vi "dfd_FXP Interpolation Simu.vi"(0 "signal in":i64[](array[numeric]), 2 "PROD2SUM":i16, 3 "init?":bool, 5 "interpolation factor":i32, 9 "coef":i64[](array[numeric]), 11 "FXPMRateSimState in":T1, 12 "#taps per phase":i32) -> (4 "signal out":i64[](array[numeric]), 15 "FXPMRateSimState out":T1)   [LabVIEW 2017, in "NI_DigFilter_FXP.lvlib"]
uses:
  <vilib>/addons/Digital Filter Design/NI_DigFilter_FXP.lvlib
  <vilib>/addons/Digital Filter Design/_Objects.llb/dfd_FXP MRate Simu State.ctl
  <vilib>/addons/Digital Filter Design/_Objects.llb/dfd_Integer I160.ctl
  <vilib>/addons/Digital Filter Design/_Objects.llb/dfd_Index Config.ctl
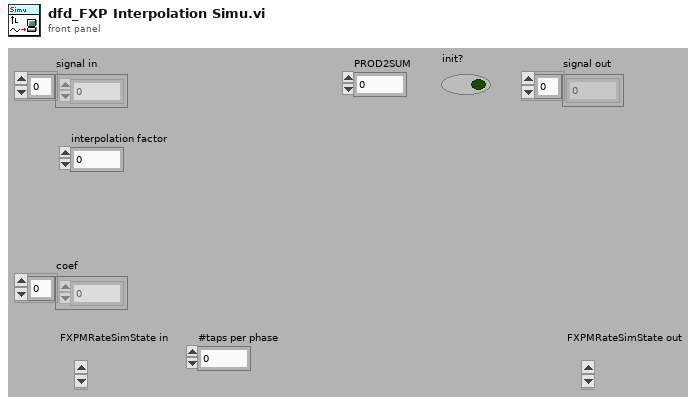
[diagram p1: front panel]
types:
  T1 = typedef "dfd_FXP MRate Simu State.ctl" = cluster{"acc1":T2[], "acc2":T2[], "FIR state":i64[], "next phase":i32}
  T2 = typedef "dfd_Integer I160.ctl" = cluster{"Hi [I32]":i32, "Lo3 [U32]":u32, "Lo2 [U32]":u32, "Lo1 [U32]":u32, "Lo0 [U32]":u32}
  T3 = typedef "dfd_Index Config.ctl" = cluster{"start":i32, "stepsize":i32}
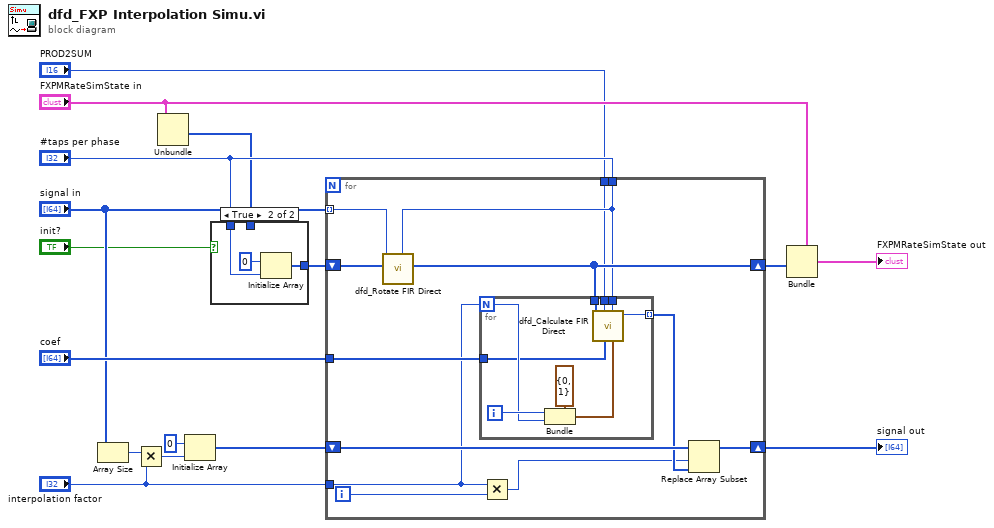
[diagram p0: block diagram]
diagram:
  n1 = Array Size(array="signal in") -> (size(s)=w11:i32)
  n2 = Multiply(x=w11, y="interpolation factor") -> (x*y=w14:i32)
  n3 = Unbundle("FXPMRateSimState in") -> ("FIR state"=w7:i64[])  [unwired: 3 out]
  n4 = Initialize Array(i64 0 ("element"), w14) -> (w12:i64[])
  n5 = case shown="True" "init?" {
    tunnel: [w17 w19] -> w8
    tunnel: "#taps per phase" -> [_ w18]
    tunnel: w7 -> [w17 _]
    frame False {
    }
    frame True {
      n6 = Initialize Array(i64 0 ("element"), w18) -> (w19:i64[])
    }
  }
  n7 = for {
    tunnel: "signal in" -> [w27] mode=indexing
    tunnel: "interpolation factor" -> [w23]
    tunnel: "#taps per phase" -> [w22]
    shift-right: [w24] -> w5
    shift-left: w8 -> [w26]
    tunnel: "coef" -> [w32]
    shift-right: [w28] -> w1
    shift-left: w12 -> [w30]
    tunnel: "PROD2SUM" -> [w21]
    i -> [w31]
    n8 = call <vilib>:"dfd_Rotate FIR Direct.vi"("#taps per phase"=w22, "state in"=w26, "x"=w27) -> ("state out"=w24:i64[])  [unwired: 1 in, 7 out]
    n9 = for {
      N: w23 -> [w35]
      tunnel: w22 -> [w38]
      tunnel: w24 -> [w36]
      tunnel: [w41] -> w29 mode=indexing
      tunnel: w32 -> [w34]
      tunnel: w21 -> [w33]
      i -> [w39]
      n10 = Bundle(cluster=T3 {"start"=0, "stepsize"=1} ("state idx"), "start"=w39, "stepsize"=w35) -> (w37:T3)
      n11 = call <vilib>:"dfd_Calculate FIR Direct.vi"("coef idx"=w37, "#taps per phase"=w38, "coef"=w34, "fwl_diff"=w33, "state in"=w36) -> ("y"=w41:i64)  [unwired: 3 in, 3 out]
    }
    n12 = Multiply(x=w23, y=w31) -> (x*y=w25:i32)
    n13 = Replace Array Subset(array=w30, new element=w29, index=w25) -> (w28:i64[])
  }
  "signal out" <- w1
  n14 = Bundle(cluster="FXPMRateSimState in", "FIR state"=w5) -> (→"FXPMRateSimState out":T1)  [unwired: 3 out]
